vi "createFiles.vi"(8 "error in (no error)":errorcluster, 11 "Log in":refnum<class "Log.lvclass">) -> (0 "error out":errorcluster, 3 "Log out":refnum<class "Log.lvclass">)   [LabVIEW 2013, in "Log.lvlib" / "Log.lvclass"]
uses:
  <userlib>/Common/Log/Log/Log.lvclass
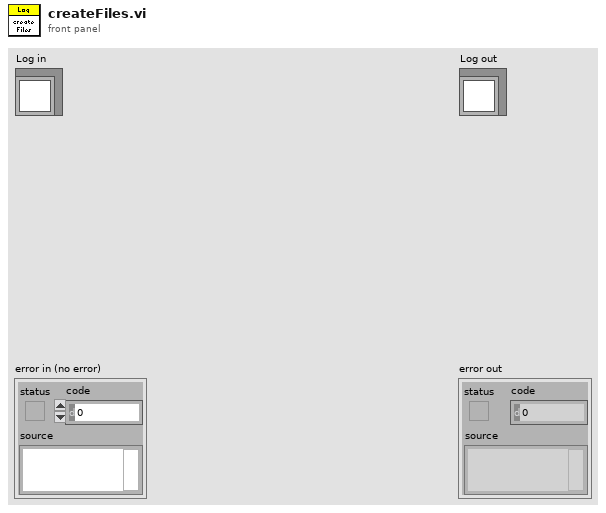
[diagram p1: front panel]
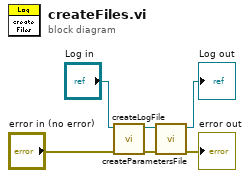
[diagram p0: block diagram]
diagram:
  n1 = call <userlib>:"createLogFile.vi"("error in (no error)"="error in (no error)", "Log in"="Log in") -> ("error out"=w3:errorcluster, "Log out"=w6:refnum<class "Log.lvclass">)  [unwired: 8 in]
  n2 = call <userlib>:"createParametersFile.vi"("error in (no error)"=w3, "Log in"=w6) -> ("error out"=→"error out":errorcluster, "Log out"=→"Log out":refnum<class "Log.lvclass">)  [unwired: 8 in]
